vi "TestEventTransport_ValueOK.vi"(8 "error in (no error)":errorcluster, 11 "TestCase in":refnum<class "TestTransport.lvclass">) -> (0 "error out":errorcluster, 3 "TestCase out":refnum<class "TestTransport.lvclass">)   [LabVIEW 2015, in "TestTransport.lvclass"]
uses:
  TestTransport.lvclass
  Framework/Mediator/Transport/EventTransport/EventTransport.lvclass
panel:
  out "element":T1
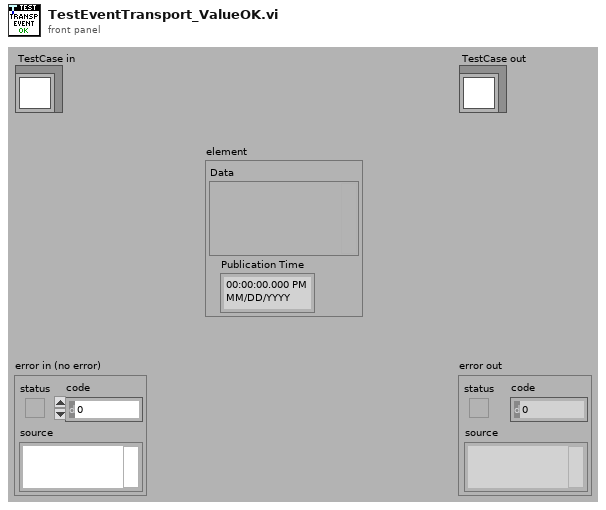
[diagram p1: front panel]
types:
  T1 = cluster{"Data":variant, "Publication Time":timestamp}
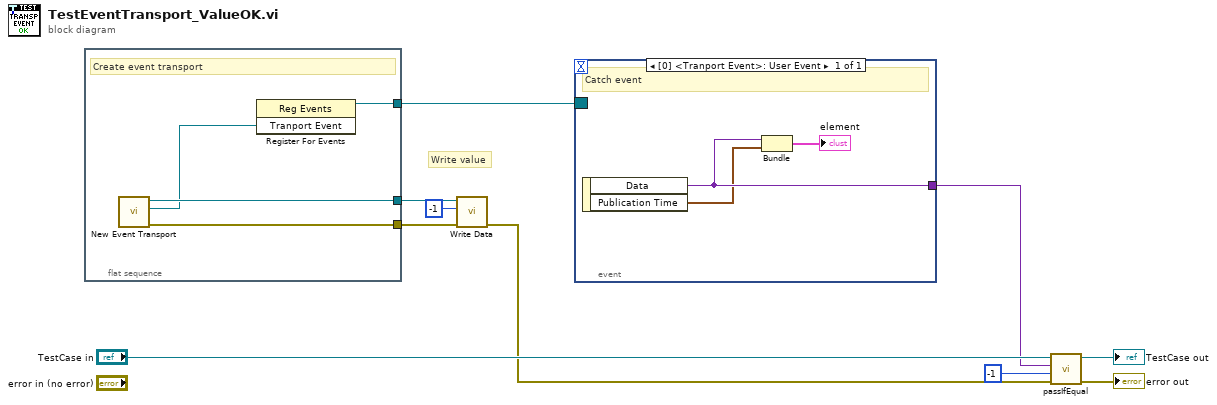
[diagram p0: block diagram]
diagram:
  # "Write value"
  n1 = flat-sequence {
    tunnel: [w14] -> w5
    tunnel: [w13] -> w4
    tunnel: [w11] -> w2
    frame #0 {
      # "Create event transport"
      n2 = call "New Event Transport.vi"() -> ("error out"=w13:errorcluster, "Tranport Event"=w12:refnum<user-event>, "EventTransport Out"=w14:refnum<class "EventTransport.lvclass">)  [unwired: 9 in]
      n3 = register-events(w12) -> (reference out=w11:refnum<event-registration>)  [unwired: 2 in, 1 out]
    }
  }
  n4 = call-dynamic "Write Data.vi"("error in (no error)"=w4, "Value"=-1, "EventTransport In"=w5) -> ("error out"=w1:errorcluster)  [unwired: 7 in, 1 out]
  n5 = event shown="[0] <Tranport Event>: User Event" {
    selector: w2 -> [_]
    dyn-events: _ -> [_]
    timeout: _ -> [_]
    tunnel: [w17] -> w3
    event User Event {
      # "Catch event"
      n6 = event-data() -> ("Data"=w17:variant, "Publication Time"=w16:timestamp)  [unwired: 1 in]
      n7 = Bundle("Data"=w17, "Publication Time"=w16) -> (→"element":T1)  [unwired: 1 in]
    }
  }
  n8 = call-dynamic "passIfEqual.vi"("error in (no error)"=w1, "y"=-1, "x"=w3, "TestCase in"="TestCase in") -> ("error out"=→"error out":errorcluster, "TestCase out"=→"TestCase out":refnum<class "TestTransport.lvclass">)  [unwired: 6 in]
